vi "init_frontpanel_controls.vi"(8 "error in":errorcluster, 10 "All frontpanel parameters":T2 {"Free run parameters"."Stim length" min=0.001 max=0.1 step=0.01; "Free run parameters"."Stim onset" min=0.0 max=100.0; "Free run parameters"."Stim frequency" min=0.1 max=40.0 step=1.0; "Device parameters"."Read chunk size" min=100 max=100000; "Device parameters"."Acquisition sample rate" min=10.0 max=10000.0 step=10.0; "Device parameters"."Stimulation sample rate" min=10.0 max=10000.0; "Protocol parameters"."Pulse width" min=0.0001 max=0.1 step=0.01; "Protocol parameters"."Acquire after ON" min=0.0 max=10.0 step=1.0; "Protocol parameters"."Acquire before ON" min=0.0 max=10.0 step=1.0; "Protocol parameters"."Repetitions" min=1.0 max=10.0 step=1.0; "Protocol parameters"."OFF time" min=0.0 max=1000.0; "Protocol parameters"."ON time" min=0.0 max=1000.0; "Protocol parameters"."Stim onset" min=0.0 max=100.0; "Protocol parameters"."Stim frequency" min=0.1 max=40.0 step=1.0}, 11 "All frontpanel references":T1) -> (0 "error out":errorcluster)   [LabVIEW 2010]
uses:
  typedefs/all_frontpanel_parameters_protocol_NI.ctl
  typedefs/run_mode.ctl
  typedefs/protocol_parameters.ctl
  typedefs/free_run_parameters.ctl
  typedefs/device_parameters.ctl
  typedefs/storage_parameters_cluster.ctl
panel:
  # "_0000.txt"
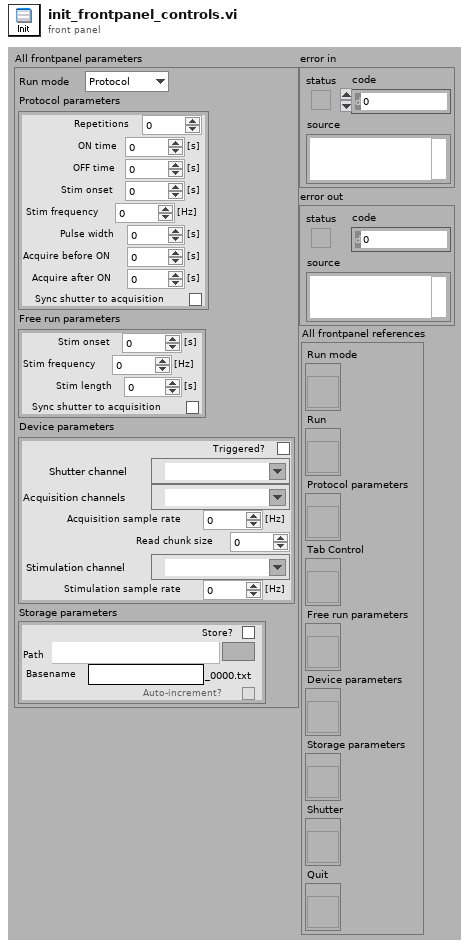
[diagram p1: front panel]
types:
  T1 = cluster{"Run mode":refnum<vi>, "Run":refnum<vi>, "Protocol parameters":refnum<vi>, "Tab Control":refnum<vi>, "Free run parameters":refnum<vi>, "Device parameters":refnum<vi>, "Storage parameters":refnum<vi>, "Shutter":refnum<vi>, "Quit":refnum<vi>}
  T2 = typedef "all_frontpanel_parameters_protocol_NI.ctl" = cluster{"Run mode":T3, "Protocol parameters":T4, "Free run parameters":T5, "Device parameters":T6, "Storage parameters":T7}
  T3 = typedef "run_mode.ctl" = enum32{"Protocol", "Free Run"}
  T4 = typedef "protocol_parameters.ctl" = cluster{"Repetitions":dbl, "ON time":dbl, "OFF time":dbl, "Stim onset":dbl, "Stim frequency":dbl, "Pulse width":dbl, "Acquire before ON":dbl, "Acquire after ON":dbl, "Sync shutter to acquisition":bool}
  T5 = typedef "free_run_parameters.ctl" = cluster{"Stim onset":dbl, "Stim frequency":dbl, "Stim length":dbl, "Sync shutter to acquisition":bool}
  T6 = typedef "device_parameters.ctl" = cluster{"Triggered?":bool, "Shutter channel":tag, "Acquisition channels":tag, "Acquisition sample rate":dbl, "Read chunk size":i32, "Stimulation channel":tag, "Stimulation sample rate":dbl}
  T7 = typedef "storage_parameters_cluster.ctl" = cluster{"Store?":bool, "Path":path, "Basename":string, "Auto-increment?":bool}
  T8 = enum32{"Protocol", "Free Run", "Storage", "Device"}
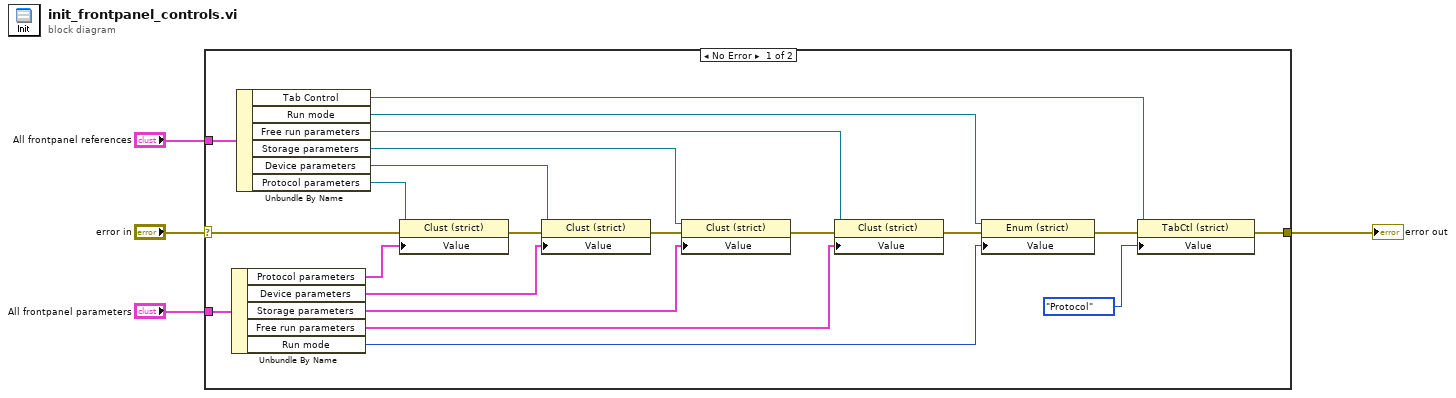
[diagram p0: block diagram]
diagram:
  n1 = case shown="No Error" "error in" {
    selector: "error in" -> [w21 w26]
    tunnel: [w5 w26] -> w3
    tunnel: "All frontpanel parameters" -> [w25 _]
    tunnel: "All frontpanel references" -> [w24 _]
    frame No Error {
      n2 = Unbundle By Name(w25) -> ("Protocol parameters"=w22:T4, "Device parameters"=w18:T6, "Storage parameters"=w15:T7, "Free run parameters"=w12:T5, "Run mode"=w9:T3)
      n3 = Unbundle By Name(w24) -> ("Tab Control"=w7:refnum<vi>, "Run mode"=w10:refnum<vi>, "Free run parameters"=w13:refnum<vi>, "Storage parameters"=w16:refnum<vi>, "Device parameters"=w19:refnum<vi>, "Protocol parameters"=w23:refnum<vi>)
      n4 = property class="Clust (strict)"(reference=w23, error in=w21, "Value"=w22) -> (error out=w20:errorcluster)  [unwired: 1 out]
      n5 = property class="Clust (strict)"(reference=w19, error in=w20, "Value"=w18) -> (error out=w17:errorcluster)  [unwired: 1 out]
      n6 = property class="Clust (strict)"(reference=w16, error in=w17, "Value"=w15) -> (error out=w14:errorcluster)  [unwired: 1 out]
      n7 = property class="Clust (strict)"(reference=w13, error in=w14, "Value"=w12) -> (error out=w11:errorcluster)  [unwired: 1 out]
      n8 = property class="Enum (strict)"(reference=w10, error in=w11, "Value"=w9) -> (error out=w8:errorcluster)  [unwired: 1 out]
      n9 = property class="TabCtl (strict)"(reference=w7, error in=w8, "Value"=T8."Protocol") -> (error out=w5:errorcluster)  [unwired: 1 out]
    }
    frame Error {
    }
  }
  "error out" <- w3
